vi "rs3 post process4.vi"(0 "Depth Input":dbl[][](graph), 1 "Color input":u8[](array[numeric]), 2 "hole fill algo":i32(ring)=1 items=["filling with left pixel", "filling with biggest of nearest pixels", "filling with smallest of nearest pixels"], 3 "Temporal Credible table":u8[](array[numeric]), 4 "Algo step":enum16{"Start", "Continue", "End", "Do Nothing"}(ring)=enum."Continue", 5 "ID":i32, 6 "downsample  parameters":T4={"focal length (pixels)"=961.0, "baseline, mm"=0.015000001, "z_units"=0.001, "Y height"=720, "X width"=1280, "Scale"=3, "Color format"=enum."RGB internal (RGB)"} {"Scale" min=1 max=8}, 7 "Time average parameters":T3={"alphaT"=0.4, "deltaDispT(1/32 disp)"=10.0}, 8 "Temporal persistence \nHole-filling":enum16{"Custom", "Default", "Max holefilling"}(ring)=enum."Default", 9 "Spatial Filter":bool=TRUE, 10 "Time Filter":bool=TRUE, 11 "Holefill":bool, 12 "Spatial filter parameters":T2={"alphaXY"=0.6, "deltaDispXY (1/32 disp)"=10.0, "iterations"=2} {"iterations" min=1 max=8; "deltaDispXY (1/32 disp)" min=0.001 max=65000; "alphaXY" min=0.001 max=1}, 16 "persistence(0=none, 8=max)":i32, 17 "transpose":bool) -> (13 "Processing time":T1={"downsample time, "=5, "temporal filter time"=0, "Spatial filter time"=0, "Back to depth time"=0, "Holefill time "=0}, 14 "Depth Output":sgl[][](graph), 15 "Color output":u8[](array[numeric]), 18 "output width":i32=428, 19 "output height":i32=240)   [LabVIEW 2017, in "libRealSense3.lvlib"]
uses:
  libRealSense3.lvlib
  realsense2ex.dll
panel:
  out "error out":errorcluster
  out "Return":u8=1
  # "RS3 Post Process"
  # "(C) Intel Corp. 2017,  AGJ"
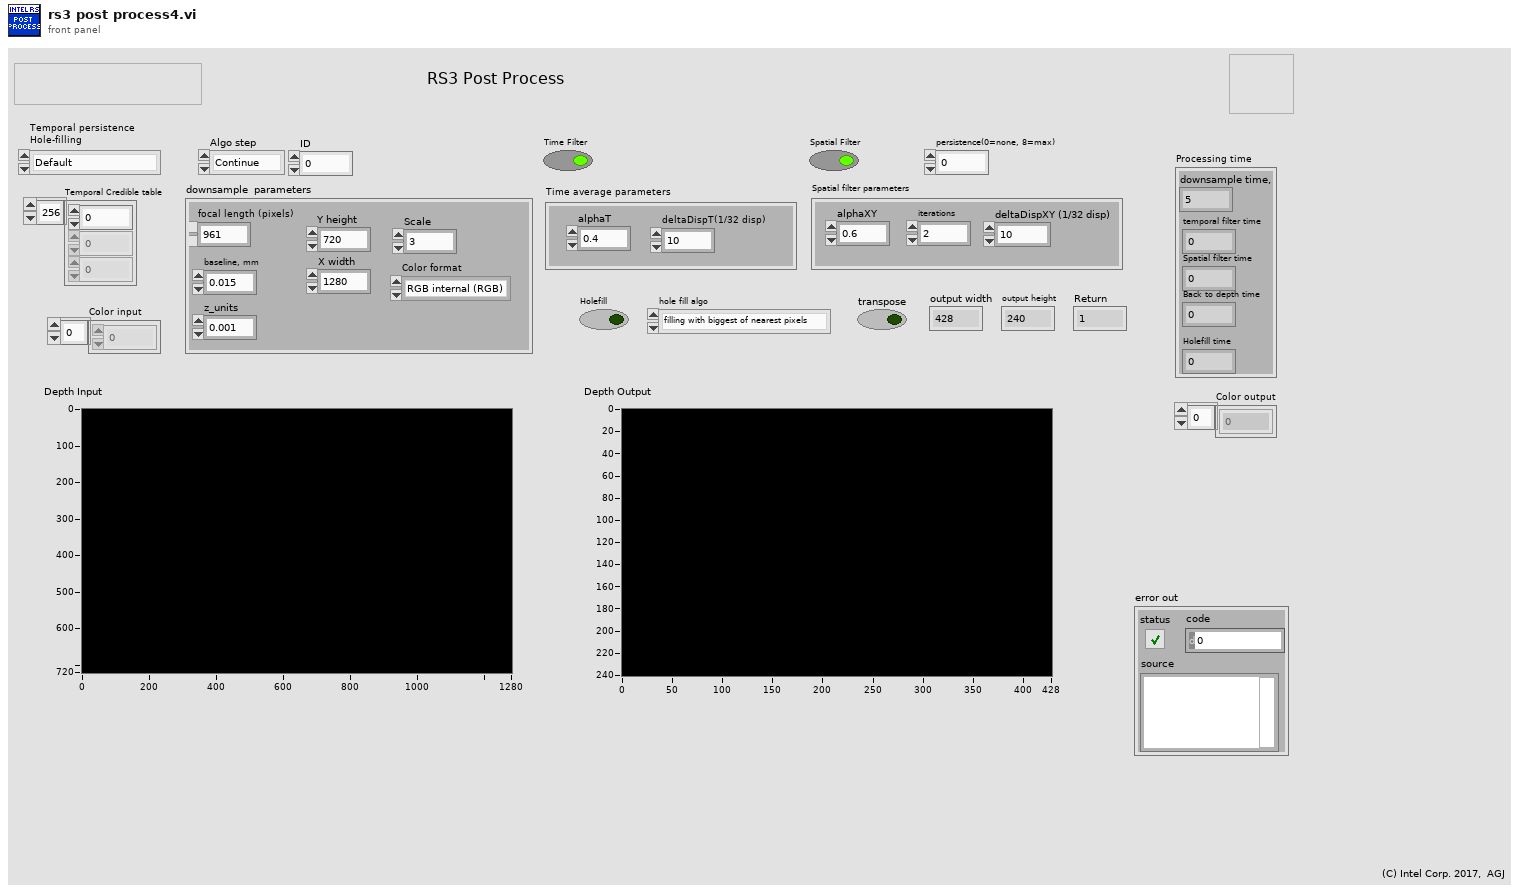
[diagram p1: front panel]
types:
  T1 = cluster{"downsample time, ":u32, "temporal filter time":u32, "Spatial filter time":u32, "Back to depth time":u32, "Holefill time ":u32}
  T2 = cluster{"alphaXY":sgl, "deltaDispXY (1/32 disp)":sgl, "iterations":i32}
  T3 = cluster{"alphaT":sgl, "deltaDispT(1/32 disp)":sgl}
  T4 = cluster{"focal length (pixels)":sgl, "baseline, mm":sgl, "z_units":sgl, "Y height":i32, "X width":i32, "Scale":i32, "Color format":enum16{"Monochrome", "RGB internal (RGB)"}}
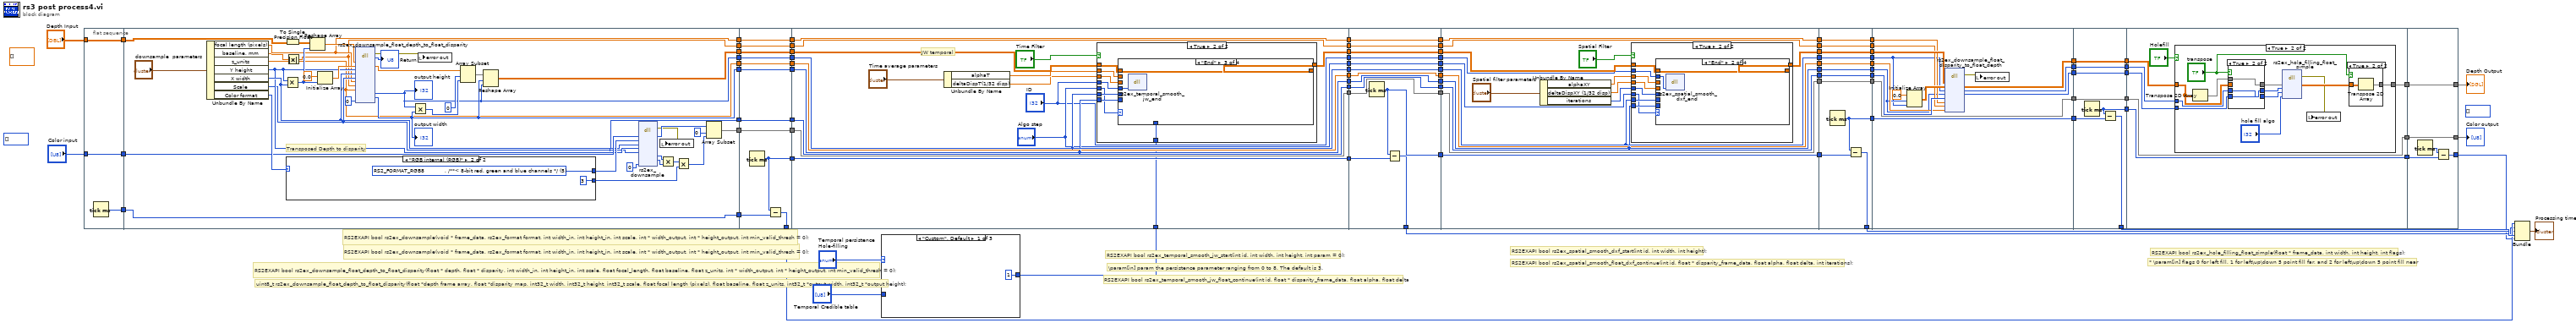
[diagram p0: block diagram]
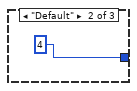
[diagram p2: hidden frame]
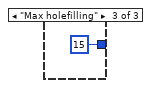
[diagram p3: hidden frame]
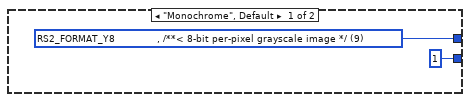
[diagram p4: hidden frame]
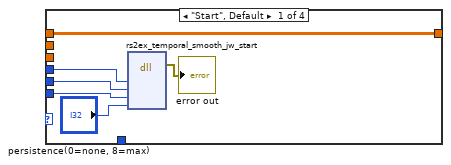
[diagram p6: hidden frame]
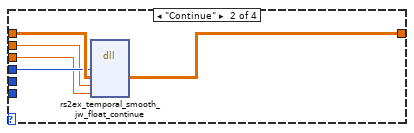
[diagram p7: hidden frame]
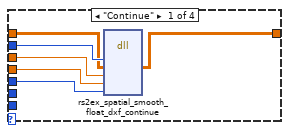
[diagram p10: hidden frame]
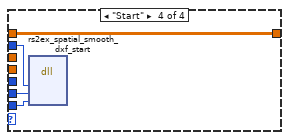
[diagram p12: hidden frame]
diagram:
  (unwired) u8[] []
  (unwired) u8[] [] ("Color input")
  (unwired) dbl[][] [] ("Depth Input")
  # "* \\param[in] flags 0 for left fill, 1 for left\\up\\down 5 point fill far, and 2 for left\\up\\down 5 point fill near"
  # "RS2EXAPI bool rs2ex_hole_filling_float_simple(float * frame_data, int width, int height, int flags);"
  # "RS2EXAPI bool rs2ex_spatial_smooth_float_dxf_continue(int id, float * disparity_frame_data, float alpha, float delta, int iterations);"
  # "RS2EXAPI bool rs2ex_spatial_smooth_dxf_start(int id, int width, int height);"
  # "RS2EXAPI bool rs2ex_temporal_smooth_jw_float_continue(int id, float * disparity_frame_data, float alpha, float delta"
  # "\\param[in] param the persistence parameter ranging from 0 to 8. The default is 3."
  # "RS2EXAPI bool rs2ex_temporal_smooth_jw_start(int id, int width, int height, int param = 0);"
  # "RS2EXAPI bool rs2ex_downsample(void * frame_data, rs2ex_format format, int width_in, int height_in, int scale, int * width_output, int * height_output, int min_valid_thresh = 0);"
  # "uint8_t rs2ex_downsample_float_depth_to_float_disparity(float *depth frame array, float *disparity map, int32_t width, int32_t height, int32_t scale, float focal length (pixels), float baseline, float z_units, int32_t *output width, int32_t *output height);"
  # "RS2EXAPI bool rs2ex_downsample_float_depth_to_float_disparity(float * depth, float * disparity, int width_in, int height_in, int scale, float focal_length, float baseline, float z_units, int * width_output, int * height_output, int min_valid_thresh = 0);"
  # "RS2EXAPI bool rs2ex_downsample(void * frame_data, rs2ex_format format, int width_in, int height_in, int scale, int * width_output, int * height_output, int min_valid_thresh = 0);"
  n1 = flat-sequence {
    tunnel: "Depth Input" -> [w89]
    tunnel: "Color input" -> [w90]
    tunnel: [w90] -> w87
    tunnel: [w89] -> w86
    tunnel: [w88] -> w66
    tunnel: w87 -> [w109]
    tunnel: w86 -> [w108]
    tunnel: [w107] -> w85
    tunnel: [w106] -> w84
    tunnel: [w100] -> w81
    tunnel: [w101] -> w79
    tunnel: [w103] -> w67
    tunnel: w66 -> [w103]
    tunnel: [w99] -> w50
    tunnel: [w98] -> w49
    tunnel: [w93] -> w38
    tunnel: [w97] -> w37
    tunnel: w85 -> [w143]
    tunnel: w84 -> [w142]
    tunnel: [w143] -> w83
    tunnel: [w142] -> w82
    tunnel: w81 -> [w141]
    tunnel: [w141] -> w80
    tunnel: w79 -> [w140]
    tunnel: [w140] -> w78
    tunnel: w67 -> [w139]
    tunnel: [w138] -> w65
    tunnel: [w137] -> w51
    tunnel: w50 -> [w137]
    tunnel: w49 -> [w136]
    tunnel: [w136] -> w48
    tunnel: [w135] -> w39
    tunnel: w38 -> [w135]
    tunnel: w37 -> [w134]
    tunnel: [w134] -> w36
    tunnel: [w133] -> w23
    tunnel: w83 -> [w156]
    tunnel: w82 -> [w160]
    tunnel: w80 -> [w154]
    tunnel: w78 -> [w153]
    tunnel: [w155] -> w77
    tunnel: [w160] -> w76
    tunnel: [w154] -> w73
    tunnel: [w153] -> w70
    tunnel: w65 -> [w152]
    tunnel: [w152] -> w64
    tunnel: [w151] -> w52
    tunnel: w51 -> [w151]
    tunnel: w48 -> [w150]
    tunnel: [w150] -> w47
    tunnel: [w149] -> w40
    tunnel: w39 -> [w149]
    tunnel: w36 -> [w148]
    tunnel: [w148] -> w35
    tunnel: ["Algo step"] -> w27
    tunnel: ["ID"] -> w18
    tunnel: w1 -> [w144]
    tunnel: w77 -> [w197]
    tunnel: w76 -> [w196]
    tunnel: [w197] -> w75
    tunnel: [w196] -> w74
    tunnel: w73 -> [w195]
    tunnel: [w195] -> w72
    tunnel: [w194] -> w71
    tunnel: w70 -> [w194]
    tunnel: w64 -> [w193]
    tunnel: [w192] -> w63
    tunnel: [w191] -> w53
    tunnel: w52 -> [w191]
    tunnel: w47 -> [w190]
    tunnel: [w190] -> w46
    tunnel: [w189] -> w41
    tunnel: w40 -> [w189]
    tunnel: w35 -> [w188]
    tunnel: [w188] -> w34
    tunnel: w27 -> [w187]
    tunnel: [w187] -> w26
    tunnel: [w186] -> w22
    tunnel: [w185] -> w19
    tunnel: w18 -> [w185]
    tunnel: w75 -> [w209]
    tunnel: w74 -> [w214]
    tunnel: w72 -> [w206]
    tunnel: w71 -> [w205]
    tunnel: [w208] -> w69
    tunnel: [w214] -> w68
    tunnel: w63 -> [w207]
    tunnel: [w207] -> w62
    tunnel: [w206] -> w58
    tunnel: [w205] -> w56
    tunnel: [w204] -> w54
    tunnel: w53 -> [w204]
    tunnel: w46 -> [w203]
    tunnel: [w203] -> w45
    tunnel: [w202] -> w42
    tunnel: w41 -> [w202]
    tunnel: w34 -> [w201]
    tunnel: [w201] -> w33
    tunnel: w26 -> [w200]
    tunnel: w19 -> [w199]
    tunnel: w69 -> [w248]
    tunnel: w68 -> [w247]
    tunnel: w62 -> [w246]
    tunnel: [w248] -> w61
    tunnel: [w247] -> w60
    tunnel: [w245] -> w59
    tunnel: w58 -> [w245]
    tunnel: [w244] -> w57
    tunnel: w56 -> [w244]
    tunnel: [w243] -> w55
    tunnel: w54 -> [w243]
    tunnel: w45 -> [w242]
    tunnel: [w242] -> w44
    tunnel: [w241] -> w43
    tunnel: w42 -> [w241]
    tunnel: w33 -> [w240]
    tunnel: [w240] -> w32
    tunnel: [w239] -> w28
    tunnel: [w238] -> w21
    tunnel: w61 -> [w262]
    tunnel: w60 -> [w263]
    tunnel: w59 -> [w254]
    tunnel: w57 -> [w255]
    tunnel: w55 -> [w259]
    tunnel: w44 -> [w258]
    tunnel: w43 -> [w257]
    tunnel: w32 -> [w256]
    tunnel: [w250] -> w31
    tunnel: [w263] -> w30
    tunnel: [w253] -> w29
    tunnel: w28 -> [w253]
    tunnel: [w252] -> w12
    tunnel: [w251] -> w10
    tunnel: w31 -> [w270]
    tunnel: w30 -> [w269]
    tunnel: w29 -> [w268]
    tunnel: [w267] -> w24
    tunnel: [w270] -> w17
    tunnel: [w269] -> w16
    tunnel: [w266] -> w13
    tunnel: w12 -> [w266]
    tunnel: [w265] -> w11
    tunnel: w10 -> [w265]
    tunnel: [w264] -> w8
    tunnel: w17 -> [w276]
    tunnel: w16 -> [w277]
    tunnel: [w275] -> w15
    tunnel: [w277] -> w14
    tunnel: w13 -> [w273]
    tunnel: w11 -> [w272]
    tunnel: [w271] -> w9
    tunnel: w8 -> [w271]
    tunnel: [w303] -> w3
    tunnel: [w304] -> w25
    tunnel: w15 -> [w304]
    tunnel: w14 -> [w303]
    tunnel: w9 -> [w301]
    tunnel: [w300] -> w7
    frame #0 {
      n2 = Tick Count (ms)() -> (millisecond timer value=w88:u32)
    }
    frame #1 {
      # "Transposed Depth to disparity"
      n3 = Unbundle By Name("downsample  parameters") -> ("focal length (pixels)"=w98:sgl, "baseline, mm"=w94:sgl, "z_units"=w97:sgl, "Y height"=w102:i32, "X width"=w104:i32, "Scale"=w99:i32, "Color format"=w112:enum16{"Monochrome", "RGB internal (RGB)"})
      n4 = Multiply(x=w102, y=w104) -> (x*y=w111:i32)
      n5 = To Single Precision Float(number=w108) -> (single precision float=w124:sgl[][])
      n6 = Absolute Value(x=w94) -> (abs(x)=w93:sgl)
      n7 = case shown="\"RGB internal (RGB)\"" w112 {
        tunnel: [w130 w132] -> w123
        tunnel: [1 ("y") 3 ("y")] -> w115
        frame "Monochrome", Default {
          w130 = u16 9 items=["    RS2_FORMAT_ANY             , /**< When passed to enable stream, librealsense will try to provide best suited format */", "    RS2_FORMAT_Z16             , /**< 16-bit linear depth values. The depth is meters is equal to depth scale * pixel value. */", "    RS2_FORMAT_DISPARITY16     , /**< 16-bit linear disparity values. The depth in meters is equal to depth scale / pixel value. */", "    RS2_FORMAT_XYZ32F          , /**< 32-bit floating point 3D coordinates. */", "    RS2_FORMAT_YUYV            , /**< Standard YUV pixel format as described in https://en.wikipedia.org/wiki/YUV */", "    RS2_FORMAT_RGB8            , /**< 8-bit red, green and blue channels */", "    RS2_FORMAT_BGR8            , /**< 8-bit blue, green, and red channels -- suitable for OpenCV */", "    RS2_FORMAT_RGBA8           , /**< 8-bit red, green and blue channels + constant alpha channel equal to FF */", "    RS2_FORMAT_BGRA8           , /**< 8-bit blue, green, and red channels + constant alpha channel equal to FF */", "    RS2_FORMAT_Y8              , /**< 8-bit per-pixel grayscale image */", "    RS2_FORMAT_Y16             , /**< 16-bit per-pixel grayscale image */", "    RS2_FORMAT_RAW10           , /**< Four 10-bit luminance values encoded into a 5-byte macropixel */", "    RS2_FORMAT_RAW16           , /**< 16-bit raw image */", "    RS2_FORMAT_RAW8            , /**< 8-bit raw image */", "    RS2_FORMAT_UYVY            , /**< Similar to the standard YUYV pixel format, but packed in a different order */", "    RS2_FORMAT_MOTION_RAW      , /**< Raw data from the motion sensor */", "    RS2_FORMAT_MOTION_XYZ32F   , /**< Motion data packed as 3 32-bit float values, for X, Y, and Z axis */", "    RS2_FORMAT_GPIO_RAW        , /**< Raw data from the external sensors hooked to one of the GPIO's */", "    RS2_FORMAT_COUNT             /**< Number of enumeration values. Not a valid input: intended to be used in for-loops. */"] ("RS Format")
        }
        frame "RGB internal (RGB)" {
          w132 = u16 5 items=["    RS2_FORMAT_ANY             , /**< When passed to enable stream, librealsense will try to provide best suited format */", "    RS2_FORMAT_Z16             , /**< 16-bit linear depth values. The depth is meters is equal to depth scale * pixel value. */", "    RS2_FORMAT_DISPARITY16     , /**< 16-bit linear disparity values. The depth in meters is equal to depth scale / pixel value. */", "    RS2_FORMAT_XYZ32F          , /**< 32-bit floating point 3D coordinates. */", "    RS2_FORMAT_YUYV            , /**< Standard YUV pixel format as described in https://en.wikipedia.org/wiki/YUV */", "    RS2_FORMAT_RGB8            , /**< 8-bit red, green and blue channels */", "    RS2_FORMAT_BGR8            , /**< 8-bit blue, green, and red channels -- suitable for OpenCV */", "    RS2_FORMAT_RGBA8           , /**< 8-bit red, green and blue channels + constant alpha channel equal to FF */", "    RS2_FORMAT_BGRA8           , /**< 8-bit blue, green, and red channels + constant alpha channel equal to FF */", "    RS2_FORMAT_Y8              , /**< 8-bit per-pixel grayscale image */", "    RS2_FORMAT_Y16             , /**< 16-bit per-pixel grayscale image */", "    RS2_FORMAT_RAW10           , /**< Four 10-bit luminance values encoded into a 5-byte macropixel */", "    RS2_FORMAT_RAW16           , /**< 16-bit raw image */", "    RS2_FORMAT_RAW8            , /**< 8-bit raw image */", "    RS2_FORMAT_UYVY            , /**< Similar to the standard YUYV pixel format, but packed in a different order */", "    RS2_FORMAT_MOTION_RAW      , /**< Raw data from the motion sensor */", "    RS2_FORMAT_MOTION_XYZ32F   , /**< Motion data packed as 3 32-bit float values, for X, Y, and Z axis */", "    RS2_FORMAT_GPIO_RAW        , /**< Raw data from the external sensors hooked to one of the GPIO's */", "    RS2_FORMAT_COUNT             /**< Number of enumeration values. Not a valid input: intended to be used in for-loops. */"] ("RS Format")
        }
      }
      n8 = Reshape Array(w124, w111) -> (w125:sgl[])
      n9 = Initialize Array(sgl 0.0 ("element"), w111) -> (w126:sgl[])
      n10 = dll-call lib="C:/Users/smartek/Desktop/labview/realsense2ex.dll" fn="rs2ex_downsample_float_depth_to_float_disparity"("depth frame array"=w125, "disparity map"=w126, "width"=w102, "height"=w104, "scale"=w99, "focal length (pixels)"=w98, "baseline"=w93, "z_units"=w97, "min valid thresh"=0) -> (error out=w95:errorcluster, "return"=→"Return":u8, "disparity map"=w113:sgl[], "output width"=w100:i32, "output height"=w101:i32)  [unwired: 13 in, 1 out]
      "output height" <- w100
      "output width" <- w101
      n11 = Multiply(x=w100, y=w101) -> (x*y=w122:i32)
      n12 = local write "error out"(w95) -> ()
      n13 = Array Subset(array=w113, index=0, length=w122) -> (w121:sgl[])
      n14 = Reshape Array(w121, w101, w100) -> (w107:sgl[][])
      n15 = dll-call lib="C:/Users/smartek/Desktop/labview/realsense2ex.dll" fn="rs2ex_downsample"("frame data pointer"=w109, "format"=w123, "width"=w104, "height"=w102, "scale"=w99, "min valid thresh"=0 ("param")) -> (error out=w96:errorcluster, "frame data pointer"=w116:u8[], "output width"=w120:i32, "output height"=w119:i32)  [unwired: 11 in, 1 out]
      n16 = local write "error out"(w96) -> ()
      n17 = Multiply(x=w120, y=w119) -> (x*y=w118:i32)
      n18 = Multiply(x=w118, y=w115) -> (x*y=w117:i32)
      n19 = Array Subset(array=w116, index=0, length=w117) -> (w106:u8[])
    }
    frame #2 {
      n20 = Tick Count (ms)() -> (millisecond timer value=w138:u32)
      n21 = Subtract(x=w138, y=w139) -> (x-y=w133:u32)
    }
    frame #3 {
      # "JW temporal"
      n22 = Unbundle By Name("Time average parameters") -> ("alphaT"=w158:sgl, "deltaDispT(1/32 disp)"=w157:sgl)
      n23 = case shown="True" "Time Filter" {
        tunnel: w158 -> [_ w170]
        tunnel: w157 -> [_ w169]
        tunnel: w156 -> [w161 w168]
        tunnel: [w161 w167] -> w155
        tunnel: w154 -> [_ w166]
        tunnel: w153 -> [_ w165]
        tunnel: "Algo step" -> [_ w164]
        tunnel: "ID" -> [_ w163]
        tunnel: w144 -> [_ w162]
        frame False {
        }
        frame True {
          n24 = case shown="\"End\"" w164 {
            tunnel: w168 -> [w176 w180 w183 w184]
            tunnel: [w176 w181 w183 w184] -> w167
            tunnel: w163 -> [w175 w179 w182 _]
            tunnel: w170 -> [_ w178 _ _]
            tunnel: w169 -> [_ w177 _ _]
            tunnel: w166 -> [w174 _ _ _]
            tunnel: w165 -> [w173 _ _ _]
            tunnel: w162 -> [_ _ _ _]
            frame "Start", Default {
              n25 = dll-call lib="C:/Users/smartek/Desktop/labview/realsense2ex.dll" fn="rs2ex_temporal_smooth_jw_start"("ID"=w175, "width"=w174, "height"=w173, "persistence"="persistence(0=none, 8=max)") -> (error out=→"error out":errorcluster)  [unwired: 8 in, 1 out]
            }
            frame "Continue" {
              n26 = dll-call lib="C:/Users/smartek/Desktop/labview/realsense2ex.dll" fn="rs2ex_temporal_smooth_jw_float_continue"("ID"=w179, "disparity 2D array"=w180, "alphaT"=w178, "deltaDispT"=w177) -> ("disparity 2D array"=w181:sgl[][])  [unwired: 7 in, 2 out]
            }
            frame "End" {
              n27 = dll-call lib="C:/Users/smartek/Desktop/labview/realsense2ex.dll" fn="rs2ex_temporal_smooth_jw_end"("ID"=w182) -> ()  [unwired: 5 in, 2 out]
            }
            frame "Do Nothing" {
            }
          }
        }
      }
    }
    frame #4 {
      n28 = Tick Count (ms)() -> (millisecond timer value=w192:u32)
      n29 = Subtract(x=w192, y=w193) -> (x-y=w186:u32)
    }
    frame #5 {
      n30 = Unbundle By Name("Spatial filter parameters") -> ("alphaXY"=w212:sgl, "deltaDispXY (1/32 disp)"=w211:sgl, "iterations"=w210:i32)
      n31 = case shown="True" "Spatial Filter" {
        tunnel: w212 -> [_ w224]
        tunnel: w211 -> [_ w223]
        tunnel: w210 -> [_ w222]
        tunnel: w209 -> [w215 w221]
        tunnel: [w215 w220] -> w208
        tunnel: w206 -> [_ w219]
        tunnel: w205 -> [_ w218]
        tunnel: w200 -> [_ w217]
        tunnel: w199 -> [_ w216]
        frame False {
        }
        frame True {
          n32 = case shown="\"End\"" w217 {
            tunnel: w219 -> [_ _ _ w237]
            tunnel: w218 -> [_ _ _ w236]
            tunnel: w216 -> [w230 w232 _ w235]
            tunnel: w224 -> [w229 _ _ _]
            tunnel: w223 -> [w228 _ _ _]
            tunnel: w222 -> [w227 _ _ _]
            tunnel: w221 -> [w226 w231 w233 w234]
            tunnel: [w225 w231 w233 w234] -> w220
            frame "Continue" {
              n33 = dll-call lib="C:/Users/smartek/Desktop/labview/realsense2ex.dll" fn="rs2ex_spatial_smooth_float_dxf_continue"("ID"=w230, "2D disparity array"=w226, "alpha"=w229, "delta"=w228, "iterations"=w227) -> ("2D disparity array"=w225:sgl[][])  [unwired: 8 in, 2 out]
            }
            frame "End" {
              n34 = dll-call lib="C:/Users/smartek/Desktop/labview/realsense2ex.dll" fn="rs2ex_spatial_smooth_dxf_end"("ID"=w232) -> ()  [unwired: 5 in, 2 out]
            }
            frame "Do Nothing" {
            }
            frame "Start" {
              n35 = dll-call lib="C:/Users/smartek/Desktop/labview/realsense2ex.dll" fn="rs2ex_spatial_smooth_dxf_start"("ID"=w235, "width"=w237, "height"=w236) -> ()  [unwired: 7 in, 2 out]
            }
          }
        }
      }
    }
    frame #6 {
      n36 = Tick Count (ms)() -> (millisecond timer value=w239:u32)
      n37 = Subtract(x=w239, y=w246) -> (x-y=w238:u32)
    }
    frame #7 {
      n38 = Initialize Array(sgl 0.0 ("element"), w255, w254) -> (w260:sgl[][])
      n39 = dll-call lib="C:/Users/smartek/Desktop/labview/realsense2ex.dll" fn="rs2ex_downsample_float_disparity_to_float_depth" label="rs2ex_downsample_float_disparity_to_depth"("disparity map input"=w262, "depth map output"=w260, "width"=w254, "height"=w255, "scale"=w259, "focal length (pixels)"=w258, "baseline"=w257, "z_unit"=w256) -> (error out=w249:errorcluster, "depth map output"=w250:sgl[][], "width"=w252:i32, "height"=w251:i32)  [unwired: 9 in, 1 out]
      n40 = local write "error out"(w249) -> ()
    }
    frame #8 {
      n41 = Tick Count (ms)() -> (millisecond timer value=w264:u32)
      n42 = Subtract(x=w264, y=w268) -> (x-y=w267:u32)
    }
    frame #9 {
      n43 = case shown="True" "Holefill" {
        tunnel: w276 -> [w278 w289]
        tunnel: [w278 w280] -> w275
        tunnel: w273 -> [_ w285]
        tunnel: w272 -> [_ w284]
        frame False {
        }
        frame True {
          n44 = Transpose 2D Array(2D array=w289) -> (transposed array=w287:sgl[][])
          n45 = case shown="True" "transpose" {
            tunnel: [w296 w299] -> w288
            tunnel: w289 -> [w296 _]
            tunnel: w287 -> [_ w299]
            tunnel: [w295 w298] -> w286
            tunnel: w285 -> [w295 w297]
            tunnel: w284 -> [w294 w298]
            tunnel: [w294 w297] -> w283
            frame False {
            }
            frame True {
            }
          }
          n46 = dll-call lib="C:/Users/smartek/Desktop/labview/realsense2ex.dll" fn="rs2ex_hole_filling_float_simple" label="rs2ex_simplehole filling"("depth map"=w288, "width"=w286, "height"=w283, "flag"="hole fill algo") -> (error out=w279:errorcluster, "depth map"=w281:sgl[][])  [unwired: 7 in, 1 out]
          n47 = local write "error out"(w279) -> ()
          n48 = case shown="True" "transpose" {
            tunnel: w281 -> [w291 w293]
            tunnel: [w291 w292] -> w280
            frame False {
            }
            frame True {
              n49 = Transpose 2D Array(2D array=w293) -> (transposed array=w292:sgl[][])
            }
          }
        }
      }
    }
    frame #10 {
      n50 = Tick Count (ms)() -> (millisecond timer value=w302:u32)
      n51 = Subtract(x=w302, y=w301) -> (x-y=w300:u32)
    }
  }
  n52 = case shown="\"Custom\", Default" "Temporal persistence \nHole-filling" {
    tunnel: "Temporal Credible table" -> [_ _ _]
    tunnel: [1 4 15] -> w1
    frame "Custom", Default {
    }
    frame "Default" {
    }
    frame "Max holefilling" {
    }
  }
  n53 = Bundle(w23, w22, w21, w24, w7) -> (→"Processing time":cluster{u32, u32, u32, u32, u32})  [unwired: 1 in]
  "Color output" <- w3
  "Depth Output" <- w25
